vi "AVS_Resistivity-Monitor.vi"() -> ()   [LabVIEW 2018]
uses:
  data/Data_Display_global.vi
  Instrument_Setup_v2.vi
panel:
  out "AVS Resistance reading":dbl format="%.2f"
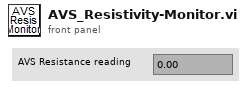
[diagram p1: front panel]
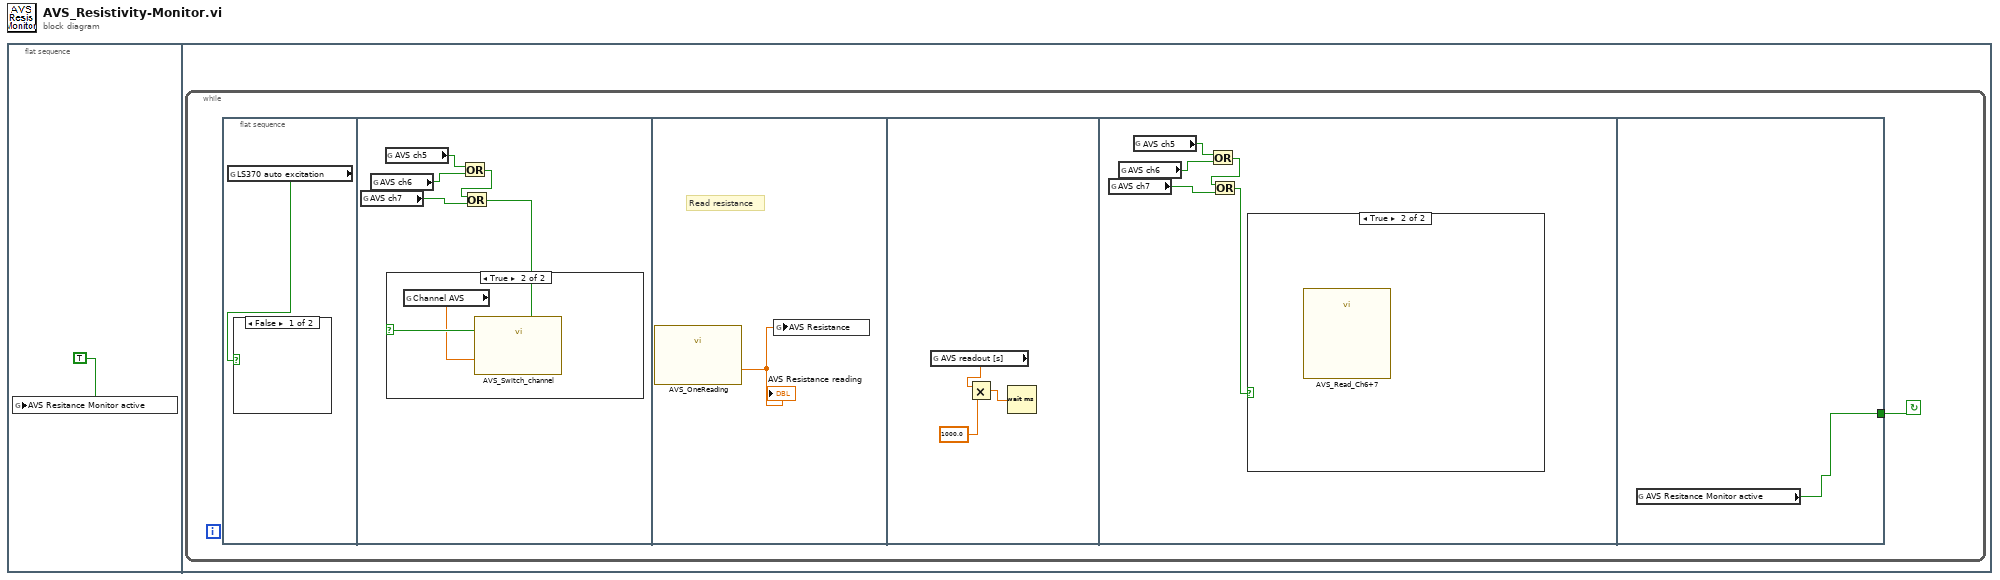
[diagram p0: block diagram]
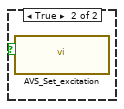
[diagram p2: hidden frame]
diagram:
  n1 = flat-sequence {
    frame #0 {
      n2 = global write "Data_Display_global.vi" "AVS Resitance Monitor active"(TRUE) -> ()
    }
    frame #1 {
      n3 = while {
        stop <- w2 continue-if-true
        n4 = flat-sequence {
          tunnel: [w19] -> w2
          frame #0 {
            n5 = global read "Data_Display_global.vi" "LS370 auto excitation"() -> (w3:bool)
            n6 = case shown="False" w3 {
              frame False {
              }
              frame True {
                n7 = call "AVS_Set_excitation.vi"() -> ()  [unwired: 12 in]
              }
            }
          }
          frame #1 {
            n8 = global read "Instrument_Setup_v2.vi" "AVS ch7"() -> (w6:bool)
            n9 = global read "Instrument_Setup_v2.vi" "AVS ch6"() -> (w7:bool)
            n10 = global read "Instrument_Setup_v2.vi" "AVS ch5"() -> (w8:bool)
            n11 = Or(x=w8, y=w7) -> (x .or. y?=w5:bool)
            n12 = Or(x=w5, y=w6) -> (x .or. y?=w4:bool)
            n13 = case shown="True" w4 {
              frame False {
              }
              frame True {
                n14 = global read "Instrument_Setup_v2.vi" "Channel AVS"() -> (w9:dbl)
                n15 = call "AVS_Switch_channel.vi"("AVS Channel"=w9) -> ()  [unwired: 11 in]
              }
            }
          }
          frame #2 {
            # "Read resistance"
            n16 = call "AVS_OneReading.vi"() -> ("AVS Resistance reading"=w10:dbl)  [unwired: 11 in]
            "AVS Resistance reading" <- w10
            n17 = global write "Data_Display_global.vi" "AVS Resistance"(w10) -> ()
          }
          frame #3 {
            n18 = global read "Instrument_Setup_v2.vi" "AVS readout [s]"() -> (w13:dbl)
            n19 = Multiply(x=w13, y=1000.0 ("AVS wait for channel [s]")) -> (x*y=w11:dbl)
            n20 = Wait (ms)(milliseconds to wait=w11) -> ()  [unwired: 1 out]
          }
          frame #4 {
            n21 = global read "Instrument_Setup_v2.vi" "AVS ch7"() -> (w14:bool)
            n22 = global read "Instrument_Setup_v2.vi" "AVS ch6"() -> (w15:bool)
            n23 = global read "Instrument_Setup_v2.vi" "AVS ch5"() -> (w16:bool)
            n24 = Or(x=w16, y=w15) -> (x .or. y?=w18:bool)
            n25 = Or(x=w18, y=w14) -> (x .or. y?=w17:bool)
            n26 = case shown="True" w17 {
              frame False {
              }
              frame True {
                n27 = call "AVS_Read_Ch6+7.vi"() -> ()  [unwired: 9 in, 3 out]
              }
            }
          }
          frame #5 {
            n28 = global read "Data_Display_global.vi" "AVS Resitance Monitor active"() -> (w19:bool)
          }
        }
      }
    }
  }
